vi "HDF5_Write_Tone_Record_20181120_b.vi"(8 "error in":errorcluster, 10 "ToneLog":T1, 11 "Cluster":T4 {"Group_ref" format="%.0x"; "Cal"."Downshift_dset" format="%.0x"; "Cal"."DeltaPhase_dset" format="%.0x"; "Cal"."Phase_dset" format="%.0x"; "Cal"."SNR_dset" format="%.0x"; "Cal"."df_dset" format="%.0x"; "Cal"."PeakLoc_dset" format="%.0x"; "Cal"."MaxValue_dset" format="%.0x"; "Cal"."TImeStamp_dset" format="%.0x"; "Cal"."TimeString_dset" format="%.0x"; "Beac"."Downshift_dset" format="%.0x"; "Beac"."DeltaPhase_dset" format="%.0x"; "Beac"."Phase_dset" format="%.0x"; "Beac"."SNR_dset" format="%.0x"; "Beac"."df_dset" format="%.0x"; "Beac"."PeakLoc_dset" format="%.0x"; "Beac"."MaxValue_dset" format="%.0x"; "Beac"."TImeStamp_dset" format="%.0x"; "Beac"."TimeString_dset" format="%.0x"; "CalZoom_dSet" format="%.0x"; "BeacZoom_dSet" format="%.0x"}) -> (0 "ErrorOut":errorcluster)   [LabVIEW 2018]
doc: "Write a single Tone<x> record with timestamp:\nTone1\n Beac - cluster\n BeacZoom - 1024 element Double array (waveform) \n Cal - cluster\n CalZoom - 1024 element Double array (waveform)"
uses:
  Controls/Clusts/ToneGroupRefsClust.ctl
  <vilib>/addons/h5labview2/base/hid_t.ctl
  HDF5_Tone_refs.ctl
  Controls/Clusts/ToneLogBuffered.ctl
  Controls/Enums/TargetNumber.ctl
  Controls/Clusts/SaturationMonitorBuffer.ctl
  <vilib>/addons/h5labview2/base/lib_path.vi
  <vilib>/addons/h5labview2/base/H5Equery.vi
  <vilib>/addons/h5labview2/dataset/H5Dwrite.llb/H5Dwrite.xnode
  <vilib>/addons/h5labview2/space/H5S.lvlib
  <vilib>/addons/h5labview2/dataset/H5D.lvlib
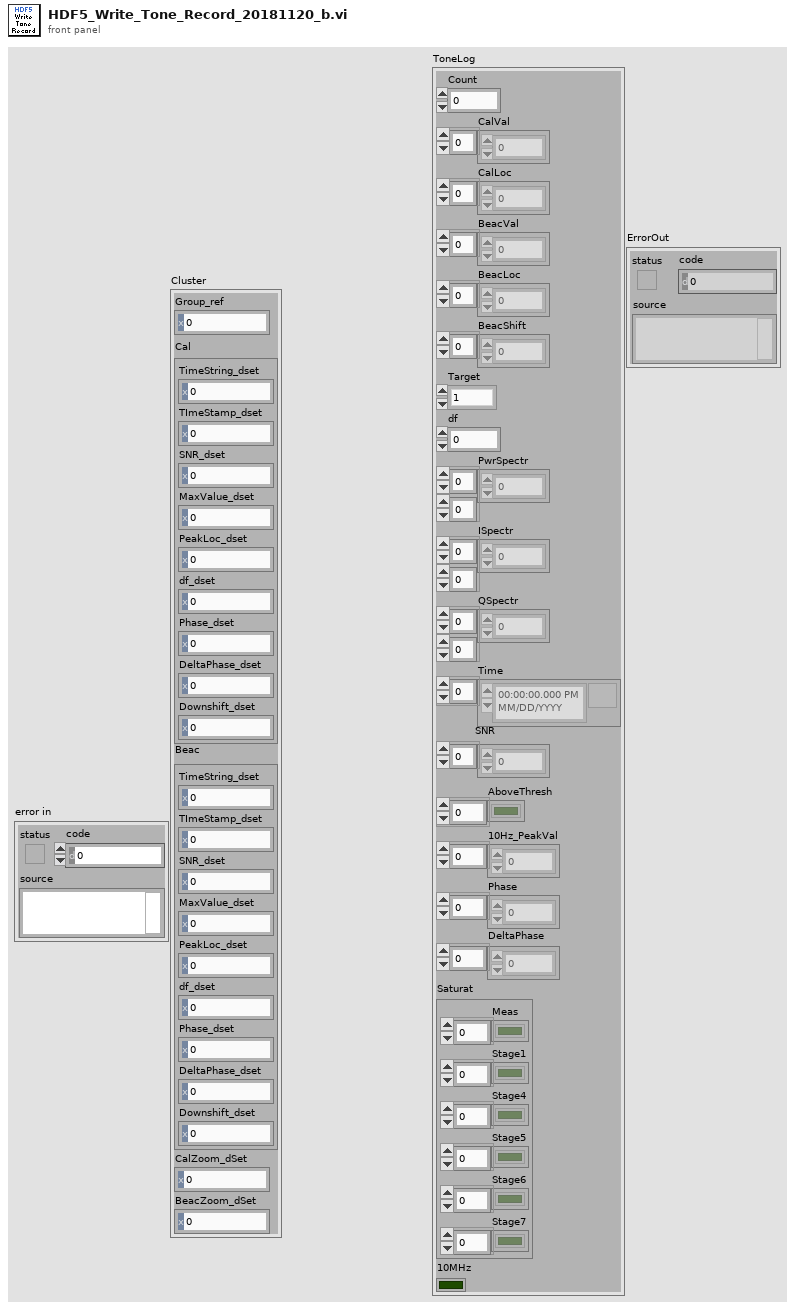
[diagram p1: front panel]
types:
  T1 = typedef "ToneLogBuffered.ctl" = cluster{"Count":i32, "CalVal":sgl[], "CalLoc":i32[], "BeacVal":sgl[], "BeacLoc":i32[], "BeacShift":i32[], "Enum":T2, "df":dbl, "PwrSpectr":sgl[][], "ISpectr":sgl[][], "QSpectr":sgl[][], "Time":timestamp[], "SNR":sgl[], "AboveThresh":bool[], "10Hz_PeakVal":dbl[], "Phase":sgl[], "DeltaPhase":dbl[], "Saturat":T3, "10MHz":bool}
  T2 = typedef "TargetNumber.ctl" = enum16{"1", "2", "3", "4"}
  T3 = typedef "SaturationMonitorBuffer.ctl" = cluster{"Meas":bool[], "Stage1":bool[], "Stage4":bool[], "Stage5":bool[], "Stage6":bool[], "Stage7":bool[]}
  T4 = typedef "ToneGroupRefsClust.ctl" = cluster{"Group_ref":T5, "Cal":T6, "Beac":T6, "CalZoom_dSet":T5, "BeacZoom_dSet":T5}
  T5 = typedef "hid_t.ctl" = i32
  T6 = typedef "HDF5_Tone_refs.ctl" = cluster{"TimeString_dset":T5, "TImeStamp_dset":T5, "SNR_dset":T5, "MaxValue_dset":T5, "PeakLoc_dset":T5, "df_dset":T5, "Phase_dset":T5, "DeltaPhase_dset":T5, "Downshift_dset":T5}
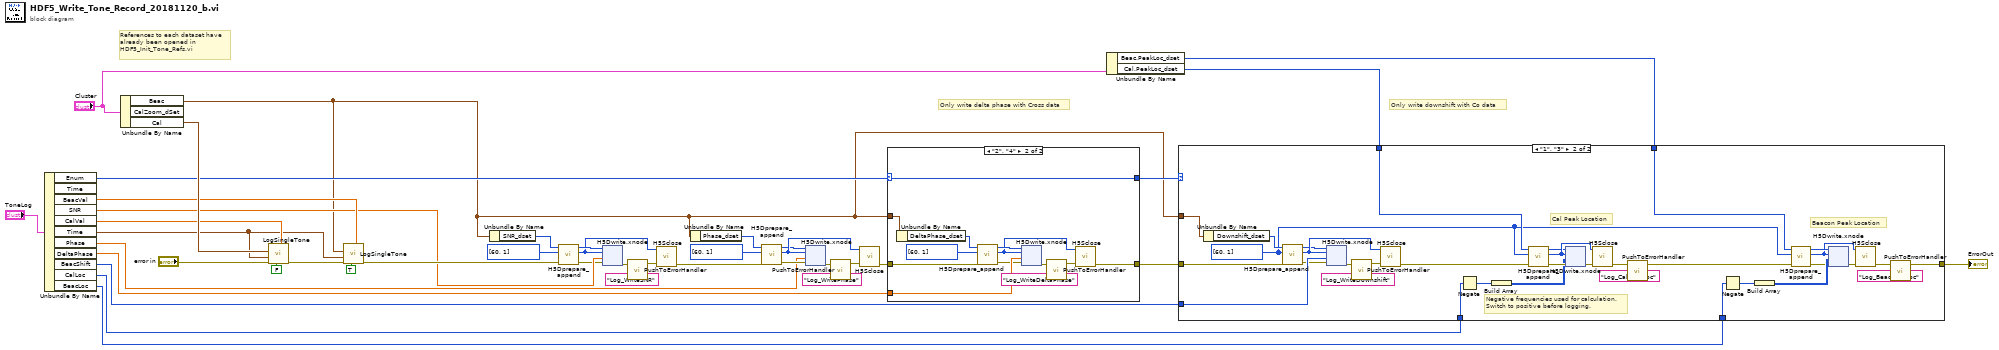
[diagram p0: block diagram]
diagram:
  # "Only write downshift with Co data"
  # "Only write delta phase with Cross data"
  # "References to each dataset have \nalready been opened in \nHDF5_Init_Tone_Refs.vi"
  n1 = Unbundle By Name("ToneLog") -> ("Enum"=w9:T2, "BeacVal"=w36:sgl[], "SNR"=w33:sgl[], "CalVal"=w35:sgl[], "Time"=w1:timestamp[], "Phase"=w13:sgl[], "DeltaPhase"=w12:dbl[], "BeacShift"=w11:i32[], "CalLoc"=w3:i32[], "BeacLoc"=w2:i32[])  [unwired: 1 out]
  n2 = Unbundle By Name("Cluster") -> ("Beac"=w7:T6, "Cal"=w41:T6)  [unwired: 1 out]
  n3 = call "LogSingleTone.vi"("MaxValue"=w35, "LogTime?"=FALSE, "error in"="error in", "seconds since 1Jan1904"=w1, "Cal"=w41) -> ("error out"=w40:errorcluster)  [unwired: 6 in]
  n4 = call "LogSingleTone.vi"("MaxValue"=w36, "LogTime?"=TRUE, "error in"=w40, "seconds since 1Jan1904"=w1, "Cal"=w7) -> ("error out"=w34:errorcluster)  [unwired: 6 in]
  n5 = Unbundle By Name(w7) -> ("SNR_dset"=w31:T5)
  n6 = call <vilib>:"H5Dprepare_append.vi"("error in (no error)"=w34, "append dims"=u64[] [60, 1], "dset in"=w31) -> ("error out"=w32:errorcluster, "space out"=w28:T5, "dset out"=w29:T5)  [unwired: 5 in, 1 out]
  n7 = xnode "H5Dwrite.xnode"("error in (no error)"=w32, "data"=w33, "file space"=w28, "ref in"=w29) -> ("error out"=w27:errorcluster)  [unwired: 3 in, 2 out]
  n8 = call "PushToErrorHandler.vi"("ErrorIn"=w27, "ErrorLocation"="Log_WriteSNR") -> ("ErrorOut"=w26:errorcluster)  [unwired: 5 in]
  n9 = call <vilib>:"H5Sclose.vi"("error in (no error)"=w26, "space in"=w28) -> ("error out"=w24:errorcluster)  [unwired: 9 in]
  n10 = Unbundle By Name(w7) -> ("Phase_dset"=w17:T5)
  n11 = call <vilib>:"H5Dprepare_append.vi"("error in (no error)"=w24, "append dims"=u64[] [60, 1], "dset in"=w17) -> ("error out"=w16:errorcluster, "space out"=w20:T5, "dset out"=w19:T5)  [unwired: 5 in, 1 out]
  n12 = xnode "H5Dwrite.xnode"("error in (no error)"=w16, "data"=w13, "file space"=w20, "ref in"=w19) -> ("error out"=w21:errorcluster)  [unwired: 3 in, 2 out]
  n13 = call "PushToErrorHandler.vi"("ErrorIn"=w21, "ErrorLocation"="Log_WritePhase") -> ("ErrorOut"=w22:errorcluster)  [unwired: 5 in]
  n14 = call <vilib>:"H5Sclose.vi"("error in (no error)"=w22, "space in"=w20) -> ("error out"=w15:errorcluster)  [unwired: 9 in]
  n15 = case shown="\"2\", \"4\"" w9 {
    selector: w9 -> [w43 w45]
    tunnel: w15 -> [w44 w57]
    tunnel: w7 -> [_ w56]
    tunnel: w12 -> [_ w55]
    tunnel: [w44 w46] -> w10
    tunnel: [w43 w45] -> w8
    frame Default {
    }
    frame "2", "4" {
      n16 = Unbundle By Name(w56) -> ("DeltaPhase_dset"=w53:T5)
      n17 = call <vilib>:"H5Dprepare_append.vi"("error in (no error)"=w57, "append dims"=u64[] [60, 1], "dset in"=w53) -> ("error out"=w54:errorcluster, "space out"=w50:T5, "dset out"=w51:T5)  [unwired: 5 in, 1 out]
      n18 = xnode "H5Dwrite.xnode"("error in (no error)"=w54, "data"=w55, "file space"=w50, "ref in"=w51) -> ("error out"=w49:errorcluster)  [unwired: 3 in, 2 out]
      n19 = call "PushToErrorHandler.vi"("ErrorIn"=w49, "ErrorLocation"="Log_WriteDeltaPhase") -> ("ErrorOut"=w48:errorcluster)  [unwired: 5 in]
      n20 = call <vilib>:"H5Sclose.vi"("error in (no error)"=w48, "space in"=w50) -> ("error out"=w46:errorcluster)  [unwired: 9 in]
    }
  }
  n21 = Unbundle By Name("Cluster") -> ("Beac.PeakLoc_dset"=w4:T5, "Cal.PeakLoc_dset"=w5:T5)
  n22 = case shown="\"1\", \"3\"" w8 {
    tunnel: [w77 w82] -> w23
    tunnel: w7 -> [_ w111]
    tunnel: w11 -> [_ w110]
    tunnel: w10 -> [w77 w102]
    tunnel: w5 -> [_ w92]
    tunnel: w4 -> [_ w81]
    tunnel: w3 -> [_ w80]
    tunnel: w2 -> [_ w79]
    frame Default {
    }
    frame "1", "3" {
      w78 = u64[] [60, 1] ("append dims")
      # "Beacon Peak Location"
      # "Cal Peak Location"
      # "Negative frequencies used for calculation.\nSwitch to positive before logging."
      n23 = Unbundle By Name(w111) -> ("Downshift_dset"=w104:T5)
      n24 = call <vilib>:"H5Dprepare_append.vi"("error in (no error)"=w102, "append dims"=w78, "dset in"=w104) -> ("error out"=w103:errorcluster, "space out"=w106:T5, "dset out"=w105:T5)  [unwired: 5 in, 1 out]
      n25 = xnode "H5Dwrite.xnode"("error in (no error)"=w103, "data"=w110, "file space"=w106, "ref in"=w105) -> ("error out"=w107:errorcluster)  [unwired: 3 in, 2 out]
      n26 = call "PushToErrorHandler.vi"("ErrorIn"=w107, "ErrorLocation"="Log_WriteDownshift") -> ("ErrorOut"=w108:errorcluster)  [unwired: 5 in]
      n27 = call <vilib>:"H5Sclose.vi"("error in (no error)"=w108, "space in"=w106) -> ("error out"=w93:errorcluster)  [unwired: 9 in]
      n28 = Negate(x=w80) -> (-x=w94:i32[])
      n29 = Build Array(w94) -> (w95:i32[][])
      n30 = call <vilib>:"H5Dprepare_append.vi"("error in (no error)"=w93, "append dims"=w78, "dset in"=w92) -> ("error out"=w97:errorcluster, "space out"=w99:T5, "dset out"=w98:T5)  [unwired: 5 in, 1 out]
      n31 = xnode "H5Dwrite.xnode"("error in (no error)"=w97, "data"=w95, "file space"=w99, "ref in"=w98) -> ("error out"=w96:errorcluster)  [unwired: 3 in, 2 out]
      n32 = call <vilib>:"H5Sclose.vi"("error in (no error)"=w96, "space in"=w99) -> ("error out"=w100:errorcluster)  [unwired: 9 in]
      n33 = call "PushToErrorHandler.vi"("ErrorIn"=w100, "ErrorLocation"="Log_CalPeakLoc") -> ("ErrorOut"=w83:errorcluster)  [unwired: 5 in]
      n34 = Negate(x=w79) -> (-x=w91:i32[])
      n35 = Build Array(w91) -> (w90:i32[][])
      n36 = call <vilib>:"H5Dprepare_append.vi"("error in (no error)"=w83, "append dims"=w78, "dset in"=w81) -> ("error out"=w88:errorcluster, "space out"=w86:T5, "dset out"=w87:T5)  [unwired: 5 in, 1 out]
      n37 = xnode "H5Dwrite.xnode"("error in (no error)"=w88, "data"=w90, "file space"=w86, "ref in"=w87) -> ("error out"=w89:errorcluster)  [unwired: 3 in, 2 out]
      n38 = call <vilib>:"H5Sclose.vi"("error in (no error)"=w89, "space in"=w86) -> ("error out"=w85:errorcluster)  [unwired: 9 in]
      n39 = call "PushToErrorHandler.vi"("ErrorIn"=w85, "ErrorLocation"="Log_BeacPeakLoc") -> ("ErrorOut"=w82:errorcluster)  [unwired: 5 in]
    }
  }
  "ErrorOut" <- w23
